vi "Check Network Connection.vi"(9 "IP Address":string, 10 "CD Path":string, 11 "connection info":T1) -> (0 "error out":errorcluster, 3 "connection info":T1)   [LabVIEW 2019, in "Control Workspace Tool.lvlib"]
uses:
  Control Workspace Tool.lvlib
  APIs/Host Automation API/Control Host Automation API.lvlib
  Workspace Shared/Control Workspace Shared.lvlib
  <vilib>/NI/STM/SubVIs/MetaDataElement.ctl
  <vilib>/NI/STM/NI STM.lvlib
  <vilib>/NI/STM/TCP/TCP Connection Info.ctl
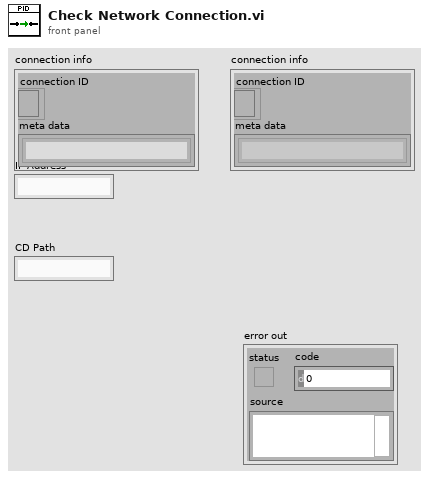
[diagram p1: front panel]
types:
  T1 = typedef "NI STM.lvlib/TCP Connection Info.ctl" = cluster{"connection ID":refnum<k5>, "meta data":T2[]}
  T2 = typedef "NI STM.lvlib/MetaDataElement.ctl" = string
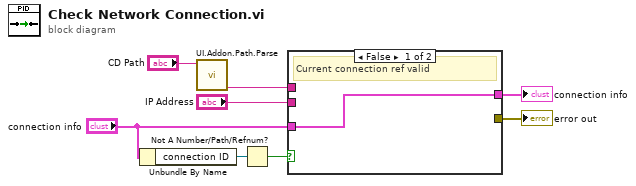
[diagram p0: block diagram]
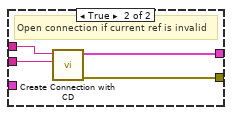
[diagram p2: hidden frame]
diagram:
  n1 = Unbundle By Name("connection info") -> ("connection ID"=w6:refnum<k5>)
  n2 = call "UI.Addon.Path.Parse.vi"("Cached Addon Path"="CD Path") -> ("Addon Name"=w1:string)  [unwired: 6 in, 4 out]
  n3 = Not A Number/Path/Refnum?(number/path/refnum=w6) -> (NaN/Path/Refnum?=w4:bool)
  n4 = case shown="False" w4 {
    tunnel: "connection info" -> [w9 _]
    tunnel: [_ w11] -> w8
    tunnel: "IP Address" -> [_ w13]
    tunnel: w1 -> [_ w12]
    tunnel: [w9 w10] -> w7
    frame False {
      # "Current connection ref valid"
    }
    frame True {
      # "Open connection if current ref is invalid"
      n5 = call "Create Connection with CD.vi"("IP Address"=w13, "TCP Service"=w12) -> ("error out"=w11:errorcluster, "connection info out"=w10:T1)  [unwired: 8 in]
    }
  }
  "error out" <- w8
  "connection info" <- w7
